vi "Reset Board.vi"(0 "GEA2 Reference In":refnum<k24>, 11 "Error In":errorcluster) -> (4 "GEA2 Reference Out":refnum<k24>, 6 "Pass/Fail?":bool, 8 "Report Text":string, 15 "Error Out":errorcluster)   [LabVIEW 2021]
doc: "Use this VI to lock or unlock the lid."
uses:
  D:/Common/LabVIEW GEA2 Toolkit/source/GEA3 DLL Source/GeaCommunication.dll
  Common/LabVIEW GEA2 Toolkit/source/GEA3 DLL Source/GeaCommunication.dll
  Common/LabVIEW GEA2 Toolkit/GEA3/type defs/Source_Destination.ctl
  Common/LabVIEW GEA2 Toolkit/GEA3/type defs/ERD Write Data In.ctl
  Common/LabVIEW GEA2 Toolkit/GEA3/type defs/Data Type.ctl
  Common/LabVIEW GEA2 Toolkit/GEA3/library/GEA2_Toolkit.lvlib
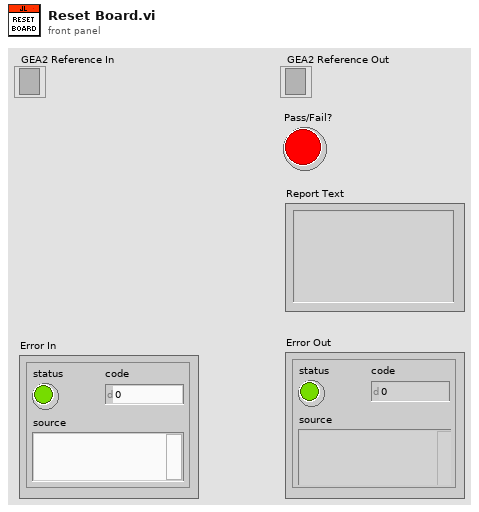
[diagram p1: front panel]
types:
  T1 = typedef "ERD Write Data In.ctl" = cluster{"ERD Number":u16, "Data Type":T2, "Data":string}
  T2 = typedef "Data Type.ctl" = enum16{"string", "boolean", "uint8_t", "uint16_t", "uint32_t", "uint64_t", "int8_t", "int16_t", "int32_t", "int64_t"}
  T3 = typedef "Source_Destination.ctl" = cluster{"Source":u8, "Destination":u8}
  T4 = cluster{"Source":u8, "Destination":u8, "Command":u8, "Length":u8, "CRC":u16, "Message":string}
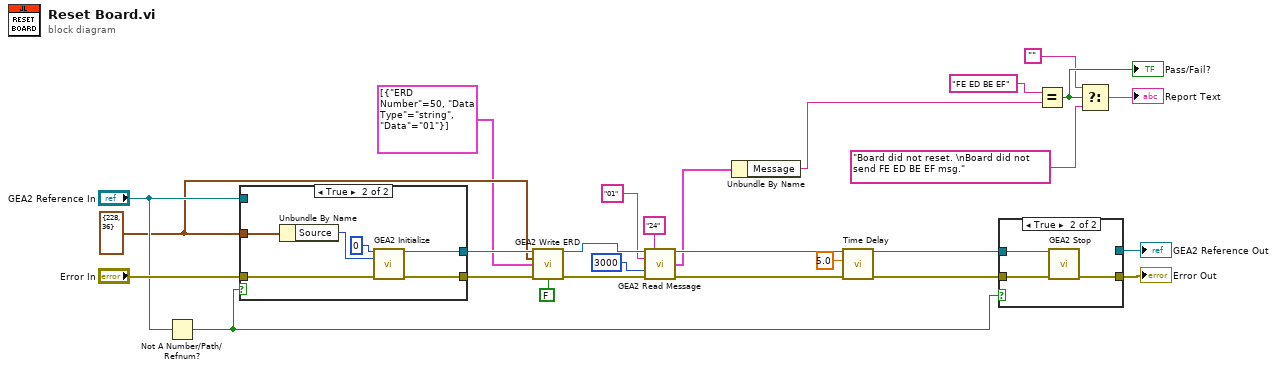
[diagram p0: block diagram]
diagram:
  w13 = T3 {"Source"=228, "Destination"=36} ("GEA Inputs")
  n1 = Not A Number/Path/Refnum?(number/path/refnum="GEA2 Reference In") -> (NaN/Path/Refnum?=w23:bool)
  n2 = case shown="True" w23 {
    tunnel: "Error In" -> [w27 w34]
    tunnel: [w27 w33] -> w17
    tunnel: "GEA2 Reference In" -> [w28 _]
    tunnel: [w28 w32] -> w15
    tunnel: w13 -> [_ w30]
    frame False {
    }
    frame True {
      n3 = Unbundle By Name(w30) -> ("Source"=w31:u8)
      n4 = call "GEA2 Initialize.vi"("Board Index"=0, "Source Address"=w31, "error in"=w34) -> ("GEA2 Reference Out"=w32:refnum<k24>, "error out"=w33:errorcluster)  [unwired: 10 in, 1 out]
    }
  }
  n5 = call "GEA2 Write ERD.vi"("GEA2 Reference In"=w15, "GEA Inputs"=w13, "Write ERD List"=T1[] [{"ERD Number"=50, "Data Type"=enum."string", "Data"="01"}], "Error In"=w17, "Verify ERD Response?"=FALSE) -> ("GEA2 Reference Out"=w14:refnum<k24>, "Error Out"=w16:errorcluster)  [unwired: 8 in, 1 out]
  n6 = call "GEA2 Read Message.vi"("GEA2 Reference In"=w14, "Expected Source"="24", "Expected Command"="01", "Timeout (ms)"=u32 3000, "Error In"=w16) -> ("GEA2 Reference Out"=w21:refnum<k24>, "Coverted Data Out"=w8:T4, "Error Out"=w3:errorcluster)  [unwired: 7 in, 1 out]
  n7 = Unbundle By Name(w8) -> ("Message"=w7:string)
  n8 = call "Time Delay"("error in (no error)"=w3, "Delay Time (s)"=5.0) -> ("error out"=w2:errorcluster)  [unwired: 9 in]
  n9 = case shown="True" w23 {
    tunnel: w2 -> [w36 w39]
    tunnel: [w36 w38] -> w26
    tunnel: [w35 _] -> w25
    tunnel: w21 -> [w35 w37]
    frame False {
    }
    frame True {
      n10 = call "GEA2 Stop.vi"("GEA2 Reference In"=w37, "Error In"=w39) -> ("Error Out"=w38:errorcluster)  [unwired: 13 in]
    }
  }
  "Error Out" <- w26
  "GEA2 Reference Out" <- w25
  n11 = Equal?(x="FE ED BE EF", y=w7) -> (x = y?=w20:bool)
  "Pass/Fail?" <- w20
  n12 = Select(t="", s=w20, f="Board did not reset. \nBoard did not send FE ED BE EF msg.") -> (s? t:f=→"Report Text":string)
